vi "Layer.vi"(7 "Activation Function":enum32{"Sigmoid", "RELU", "Tanh", "Leaky RELU"}(radio), 9 "Biases":dbl[](array[numeric]), 10 "Weights":dbl[][](array[numeric]), 11 "Data":dbl[](array[numeric])) -> (0 "Error":i32, 2 "Net Activation":dbl[](array[numeric]), 3 "Output":dbl[](array[numeric]))   [LabVIEW 2019]
uses:
  Globals.vi
  <vilib>/Analysis/NI_AALBase.lvlib
  <vilib>/Analysis/baseanly.llb/A x Vector.vi
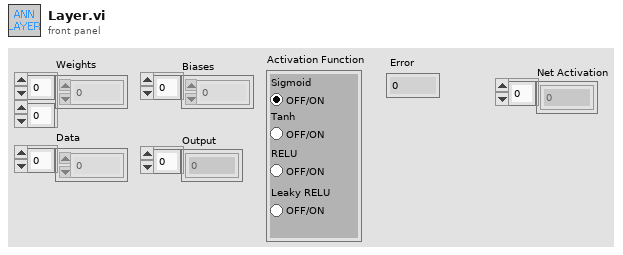
[diagram p1: front panel]
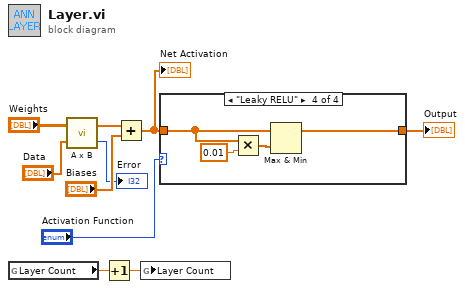
[diagram p0: block diagram]
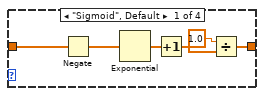
[diagram p2: hidden frame]
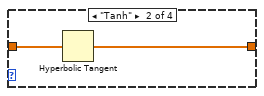
[diagram p3: hidden frame]
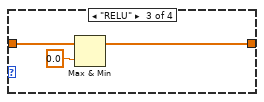
[diagram p4: hidden frame]
diagram:
  n1 = global read "Globals.vi" "Layer Count"() -> (w6:dbl)
  n2 = call-poly <vilib>:"A x B.vi"("Vector"="Data", "A"="Weights") -> ("error"=→"Error":i32, "A x Vector"=w2:dbl[])
  n3 = Increment(x=w6) -> (x+1=w5:dbl)
  n4 = Add(x=w2, y="Biases") -> (x+y=w7:dbl[])
  "Net Activation" <- w7
  n5 = global write "Globals.vi" "Layer Count"(w5) -> ()
  n6 = case shown="\"Leaky RELU\"" "Activation Function" {
    tunnel: [w11 w17 w19 w22] -> w8
    tunnel: w7 -> [w12 w18 w20 w23]
    frame "Sigmoid", Default {
      n7 = Negate(x=w12) -> (-x=w14:dbl[])
      n8 = Exponential(1:w14) -> (0:w13:dbl[])
      n9 = Increment(x=w13) -> (x+1=w15:dbl[])
      n10 = Divide(x=1.0, y=w15) -> (x/y=w11:dbl[])
    }
    frame "Tanh" {
      n11 = Hyperbolic Tangent(1:w18) -> (0:w17:dbl[])
    }
    frame "RELU" {
      n12 = Max & Min(x=w20, y=0.0) -> (max(x,y)=w19:dbl[])  [unwired: 1 out]
    }
    frame "Leaky RELU" {
      n13 = Multiply(x=w23, y=0.01) -> (x*y=w25:dbl[])
      n14 = Max & Min(x=w23, y=w25) -> (max(x,y)=w22:dbl[])  [unwired: 1 out]
    }
  }
  "Output" <- w8
